vi "Set Selected Group.vi"(8 "error in (no error)":errorcluster, 10 "Selected Group":T1, 11 "Cfg Grandmaster in":refnum<class "Cfg Grandmaster.lvclass">) -> (0 "error out":errorcluster, 3 "Cfg Grandmaster out":refnum<class "Cfg Grandmaster.lvclass">)   [LabVIEW 2018, in "Configuration Grandmaster.lvlib" / "Cfg Grandmaster.lvclass"]
uses:
  Cfg Grandmaster.lvclass
  Common/Controls/Selected Group.ctl
  Common/Controls/TE_Designator.ctl
  Cfg Grandmaster.lvclass/Cfg Grandmaster.ctl
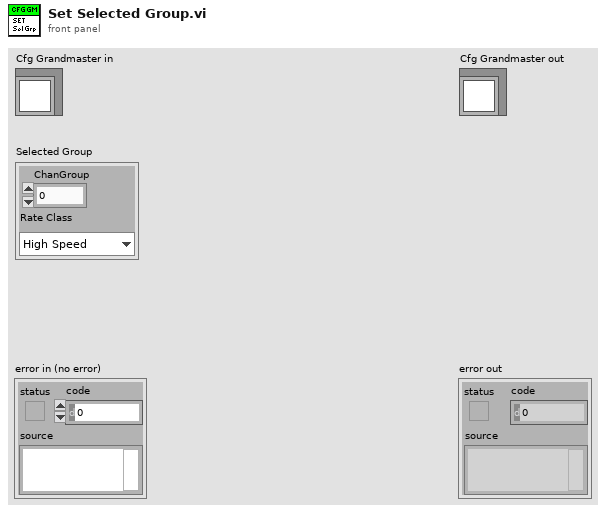
[diagram p1: front panel]
types:
  T1 = typedef "Selected Group.ctl" = cluster{"ChanGroup":i32, "Rate Class":T2}
  T2 = typedef "TE_Designator.ctl" = enum16{"High Speed", "Low Speed"}
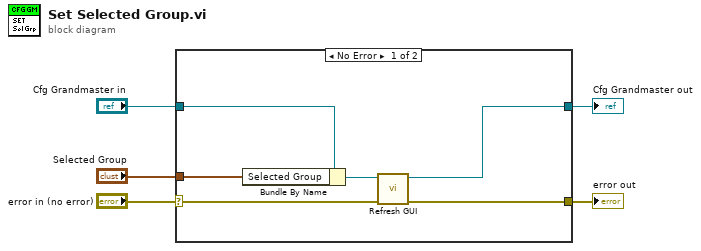
[diagram p0: block diagram]
diagram:
  n1 = case shown="No Error" "error in (no error)" {
    selector: "error in (no error)" -> [w9 w13]
    tunnel: [w8 w13] -> w4
    tunnel: [w6 w12] -> w2
    tunnel: "Cfg Grandmaster in" -> [w11 w12]
    tunnel: "Selected Group" -> [w10 _]
    frame No Error {
      n2 = Bundle By Name(cluster=w11, "Selected Group"=w10) -> (w7:refnum<class "Cfg Grandmaster.lvclass">)
      n3 = call "Refresh GUI.vi"("error in (no error)"=w9, "Cfg Grandmaster in"=w7) -> ("error out"=w8:errorcluster, "Cfg Grandmaster out"=w6:refnum<class "Cfg Grandmaster.lvclass">)  [unwired: 8 in]
    }
    frame Error {
    }
  }
  "error out" <- w4
  "Cfg Grandmaster out" <- w2
